vi "Unit Test - Standardize CSM Module.vi"() -> (0 "error out":errorcluster)   [LabVIEW 2017, in "testcase-csmhelper.lvclass"]
uses:
  testcase-csmhelper.lvclass
  src/user.lib/_NEVSTOP/Communicable State Machine(CSM)/_csmHelper/API/Create From VI Reference.vi
  src/user.lib/_NEVSTOP/Communicable State Machine(CSM)/_csmHelper/API/Open Block Diagram.vi
  src/user.lib/_NEVSTOP/Communicable State Machine(CSM)/_csmHelper/API/Destroy.vi
  src/user.lib/_NEVSTOP/Communicable State Machine(CSM)/_csmHelper/CSM-Helper.lvclass
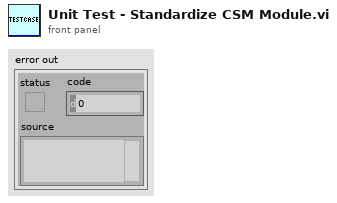
[diagram p1: front panel]
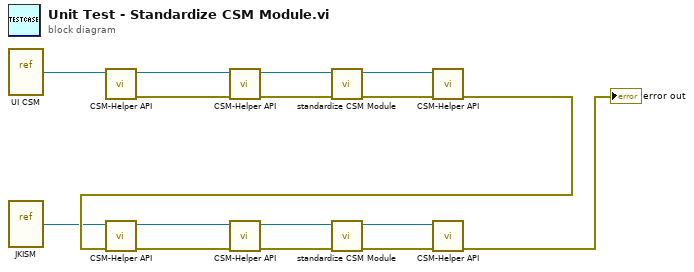
[diagram p0: block diagram]
diagram:
  n1 = vi-ref "UI CSM.vi"() -> (w16:refnum<vi>)
  n2 = vi-ref "JKISM.vi"() -> (w1:refnum<vi>)
  n3 = call-poly "CSM-Helper API.vi"("VI"=w16) -> ("error out"=w12:errorcluster, "CSM-Helper.lvclass"=w13:refnum<class "CSM-Helper.lvclass">)  [unwired: 9 in]
  n4 = call-poly "CSM-Helper API.vi"("error in (no error)"=w12, "CSM-Helper in"=w13) -> ("error out"=w11:errorcluster, "CSM-Helper out"=w10:refnum<class "CSM-Helper.lvclass">)  [unwired: 8 in]
  n5 = call "standardize CSM Module.vi"("error in"=w11, "CSM-Helper in"=w10) -> ("error out"=w15:errorcluster, "CSM-Helper out"=w14:refnum<class "CSM-Helper.lvclass">)  [unwired: 8 in]
  n6 = call-poly "CSM-Helper API.vi"("error in (no error)"=w15, "CSM-Helper in"=w14) -> ("error out"=w9:errorcluster)  [unwired: 8 in, 1 out]
  n7 = call-poly "CSM-Helper API.vi"("error in (no error)"=w9, "VI"=w1) -> ("error out"=w5:errorcluster, "CSM-Helper.lvclass"=w4:refnum<class "CSM-Helper.lvclass">)  [unwired: 8 in]
  n8 = call-poly "CSM-Helper API.vi"("error in (no error)"=w5, "CSM-Helper in"=w4) -> ("error out"=w6:errorcluster, "CSM-Helper out"=w7:refnum<class "CSM-Helper.lvclass">)  [unwired: 8 in]
  n9 = call "standardize CSM Module.vi"("error in"=w6, "CSM-Helper in"=w7) -> ("error out"=w2:errorcluster, "CSM-Helper out"=w3:refnum<class "CSM-Helper.lvclass">)  [unwired: 8 in]
  n10 = call-poly "CSM-Helper API.vi"("error in (no error)"=w2, "CSM-Helper in"=w3) -> ("error out"=→"error out":errorcluster)  [unwired: 8 in, 1 out]
